vi "Get Current PV.vi"(8 "error in":errorcluster, 11 "VISA resource name":refnum<visa-resource-name>) -> (0 "error out":errorcluster, 2 "Current PV":dbl, 3 "VISA resource name out":refnum<visa-resource-name>, 5 "Data Valid":bool)   [LabVIEW 2015, in "Samwontech TEMP2xxx.lvlib"]
doc: "Read current presented value (Symbol: NPV)\nValue stored in D0001 register"
uses:
  Samwontech TEMP2xxx.lvlib
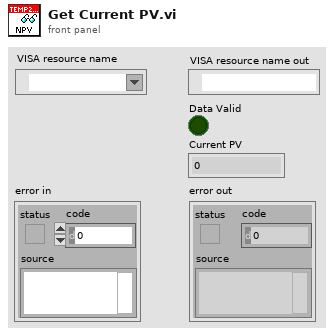
[diagram p1: front panel]
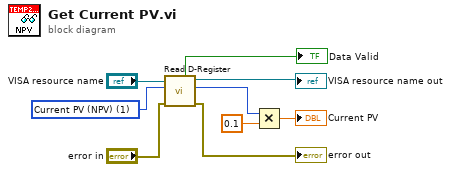
[diagram p0: block diagram]
diagram:
  w1 = u32 1 items=["Current PV (NPV)"=1, "Operation Control (COM.OPMODE)"=102, "Set Point on FIX operation (FIX.TSP)"=104, "Operation Mode (OP.MODE)"=106] ("D-Registers Map")
  n1 = call "Read D-Register.vi"("error in"="error in", "D-register number"=w1, "VISA resource name"="VISA resource name") -> ("error out"=→"error out":errorcluster, "Data"=w4:i16, "VISA resource name out"=→"VISA resource name out":refnum<visa-resource-name>, "Data Valid"=→"Data Valid":bool)  [unwired: 4 in, 1 out]
  n2 = Multiply(x=w4, y=0.1) -> (x*y=→"Current PV":dbl)
